vi "Send.vi"(8 "error in (no error)":errorcluster, 10 "Message":refnum<class "MSG.lvclass">, 11 "EventMessenger in":refnum<class "EventMessenger.lvclass">) -> (0 "error out":errorcluster, 3 "EventMessenger out":refnum<class "EventMessenger.lvclass">)   [LabVIEW 2011, in "Messenging.lvlib" / "EventMessenger.lvclass"]
uses:
  EventMessenger.lvclass
  Messenger (Parent)/MGR.lvclass
  TextVarientMessage/MSG.lvclass
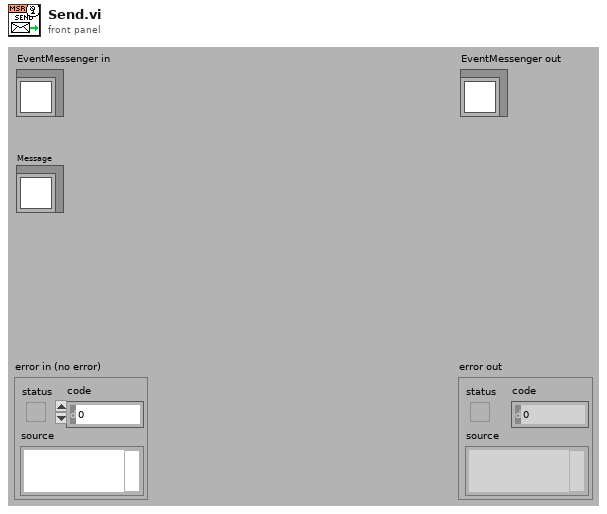
[diagram p1: front panel]
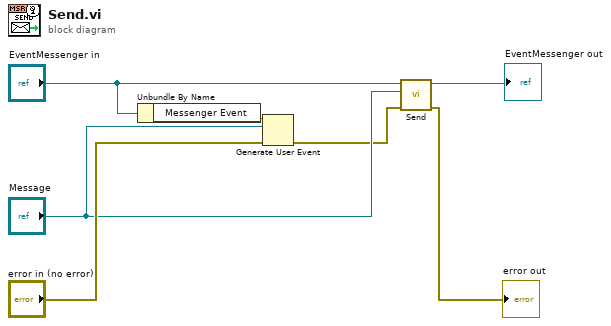
[diagram p0: block diagram]
diagram:
  n1 = Unbundle By Name("EventMessenger in") -> ("Messenger Event"=w7:refnum<user-event>)
  n2 = Generate User Event(user event=w7, event data cluster="Message", error in="error in (no error)") -> (error out=w2:errorcluster)  [unwired: 1 out]
  n3 = call-parent "Send.vi"("error in (no error)"=w2, "Message"="Message", "MSR Parent in"="EventMessenger in") -> ("error out"=→"error out":errorcluster, "MSR Parent out"=→"EventMessenger out":refnum<class "EventMessenger.lvclass">)  [unwired: 7 out]
